vi "Apply Style - button.vi"(6 "button ref":refnum<vi>, 8 "error in":errorcluster, 11 "Theme in":refnum<class "Theme.lvclass">) -> (0 "error out":errorcluster, 3 "Theme out":refnum<class "Theme.lvclass">)   [LabVIEW 2021, in "Theme.lvclass"]
doc: "Apply the theme style to a button (colors)\n\n<b>Code Developed By:</b>\nTechnology Service Corporation\n1983 S Liberty Drive\nBloomington, IN 47403\nPhone: 812 558-7100\nwww.tsc.com/atcs\n\nDeveloper:\nDaniel Coons"
uses:
  Theme.lvclass
  Theme.lvclass/Theme.ctl
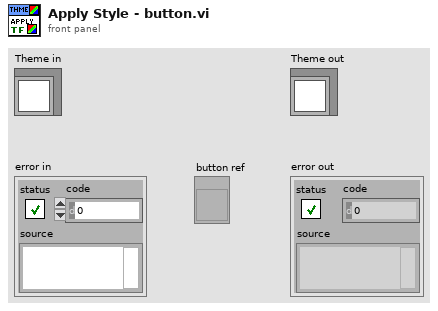
[diagram p1: front panel]
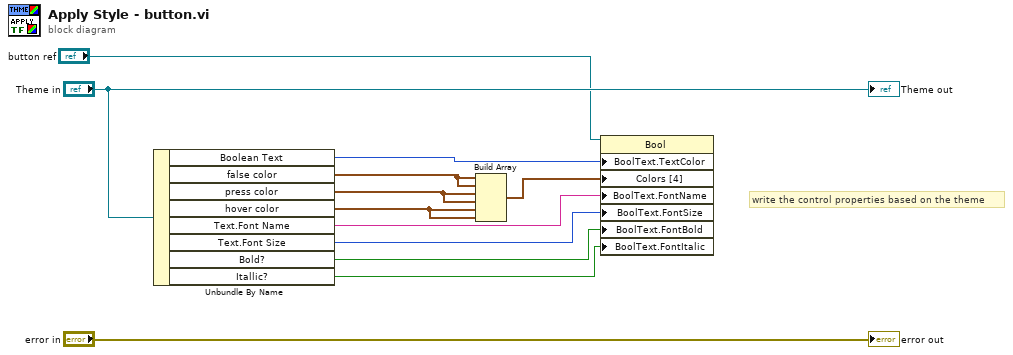
[diagram p0: block diagram]
diagram:
  # "write the control properties based on the theme"
  n1 = Unbundle By Name("Theme in") -> ("Boolean Text"=w9:u32, "false color"=w8:cluster{"border":u32, "fill":u32}, "press color"=w7:cluster{"border":u32, "fill":u32}, "hover color"=w6:cluster{"border":u32, "fill":u32}, "Text.Font Name"=w4:string, "Text.Font Size"=w3:u32, "Bold?"=w1:bool, "Itallic?"=w2:bool)
  n2 = Build Array(w8, w8, w7, w7, w6, w6) -> (w5:cluster{"border":u32, "fill":u32}[])
  n3 = property on="Property Node" class="Bool"(reference="button ref", "BoolText.TextColor"=w9, "Colors [4]"=w5, "BoolText.FontName"=w4, "BoolText.FontSize"=w3, "BoolText.FontBold"=w1, "BoolText.FontItalic"=w2) -> ()  [unwired: 1 in, 2 out]
  "error out" <- "error in"
  "Theme out" <- "Theme in"
